vi "Choreo_DifferentialSample_Interpolate.vi"(9 "TimeStamp":dbl, 10 "endValueSample":T1={"timestamp"=-999.0, "x"=0.0, "y"=0.0, "heading"=0.0, "velocityL"=0.0, "velocityR"=0.0, "angularVelocity"=0.0, "accelL"=0.0, "accelR"=0.0, "accelAngular"=0.0, "forceL"=0.0, "forceR"=0.0}, 11 "ChoreoDifferentialSample":T1={"timestamp"=-999.0, "x"=0.0, "y"=0.0, "heading"=0.0, "velocityL"=0.0, "velocityR"=0.0, "angularVelocity"=0.0, "accelL"=0.0, "accelR"=0.0, "accelAngular"=0.0, "forceL"=0.0, "forceR"=0.0}) -> (3 "InterpolatedSample":T1={"timestamp"=-999.0, "x"=0.0, "y"=0.0, "heading"=0.0, "velocityL"=0.0, "velocityR"=0.0, "angularVelocity"=0.0, "accelL"=0.0, "accelR"=0.0, "accelAngular"=0.0, "forceL"=0.0, "forceR"=0.0})   [LabVIEW 2019, in "ChoreoLib.lvlib"]
doc: "Interpolate between two Differential Trajectory Samples.\n\nInputs:\n -- ChoreoDifferentialSample - cluster - Differential sample.\n -- endChoreoDifferentialSample - cluster - The end Differential sample\n -- TimeStamp - double - desired time stamp\n\nOutputs:\n -- InterpolatedSample - cluster - Interpolated Differential sample."
uses:
  ChoreoLib.lvlib
  TypeDef/ChoreoDifferentialSample.ctl
  <vilib>/Rock Robotics/WPI/ThirdParty/JAS_Junk/TrajLib/MathUtil_Clamp.vi
  Choreo_DifferentialSample_IntegrateFunction.vi
  <vilib>/Rock Robotics/WPI/ThirdParty/JAS_Junk/TrajLib/Trajectory_Library.lvlib
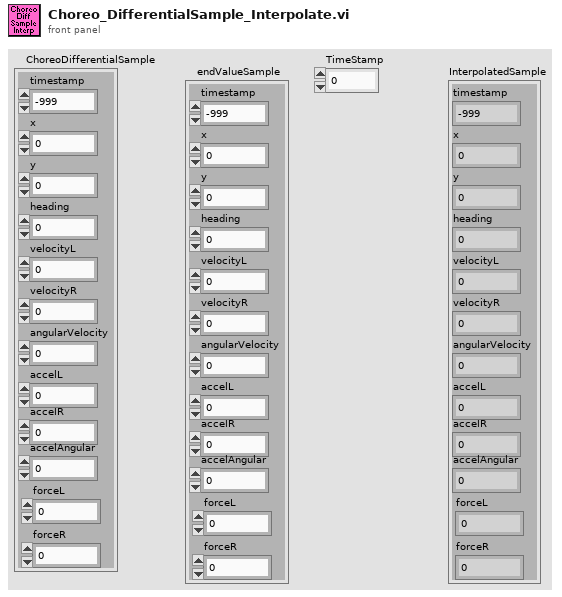
[diagram p1: front panel]
types:
  T1 = typedef "ChoreoLib.lvlib/ChoreoDifferentialSample.ctl" = cluster{"timestamp":dbl, "x":dbl, "y":dbl, "heading":dbl, "velocityL":dbl, "velocityR":dbl, "angularVelocity":dbl, "accelL":dbl, "accelR":dbl, "accelAngular":dbl, "forceL":dbl, "forceR":dbl}
  T2 = typedef "NI_Matrix.lvlib/RealMatrix.ctl" = dbl[][]
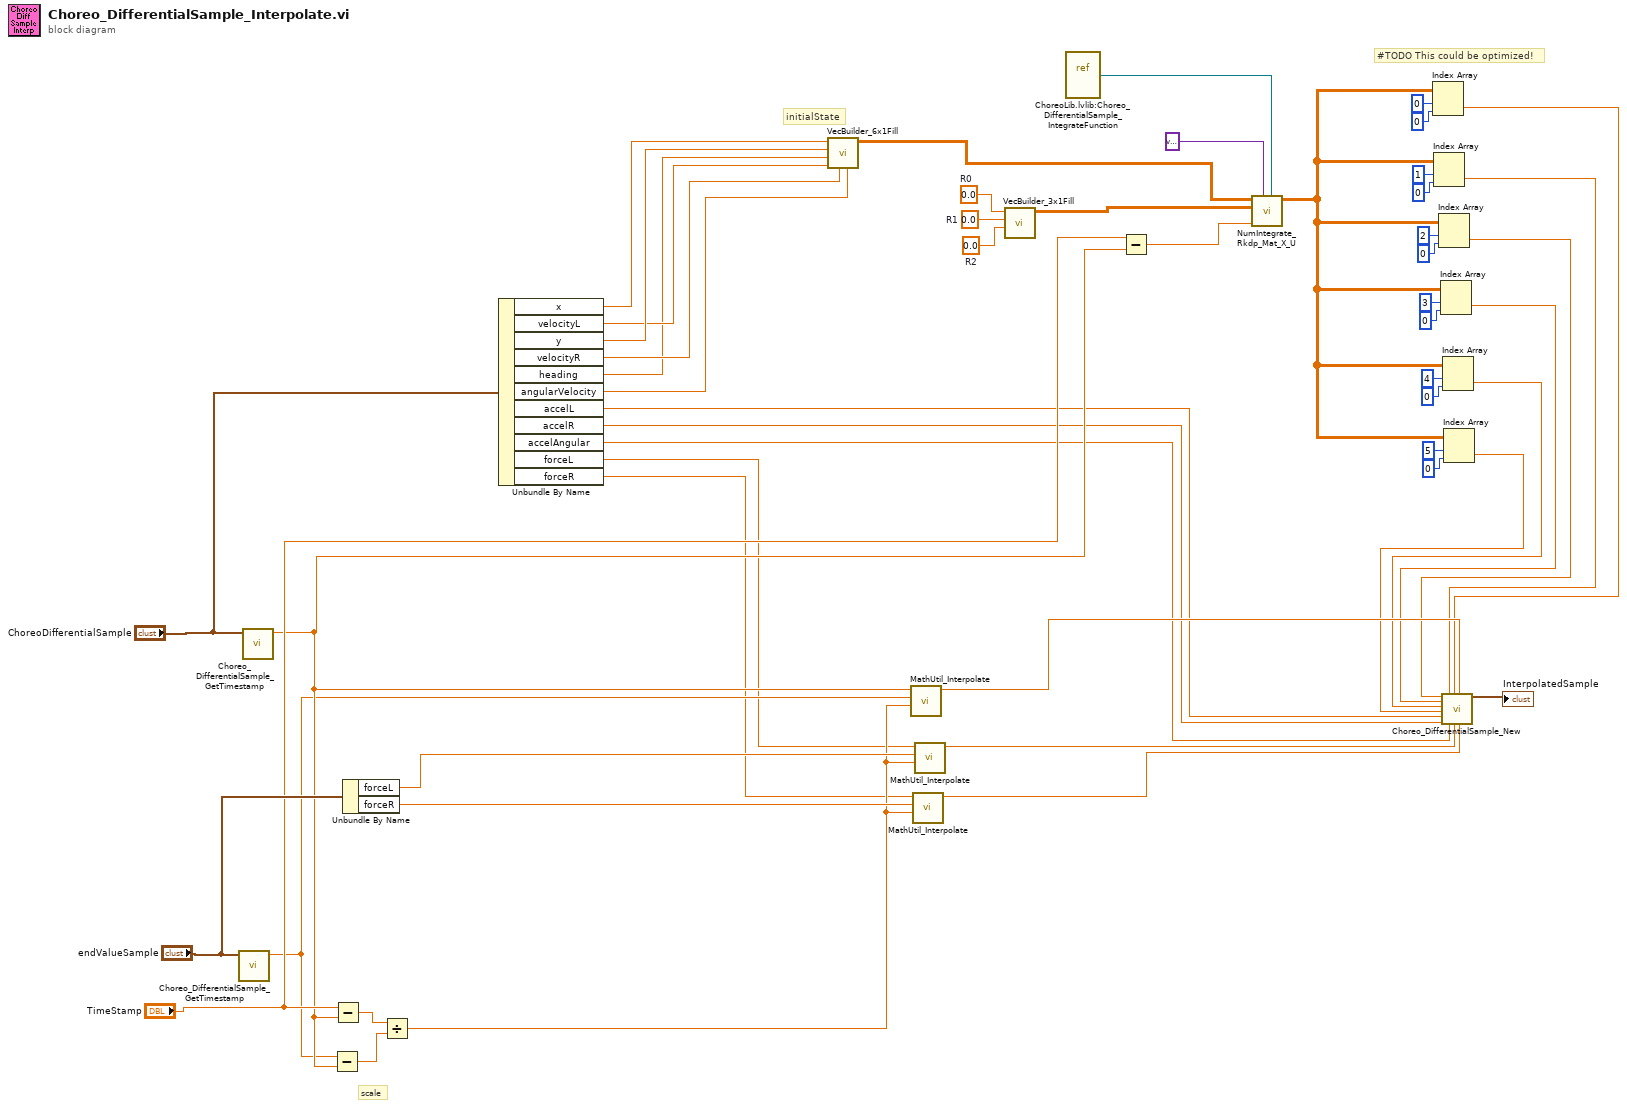
[diagram p0: block diagram]
diagram:
  w35 = 0.0  # R2
  w34 = 0.0  # R1
  w33 = 0.0  # R0
  # "#TODO This could be optimized!"
  # "initialState"
  # "scale"
  n1 = call "Choreo_DifferentialSample_GetTimestamp.vi"("ChoreoDifferentialSample"="endValueSample") -> ("Timestamp"=w28:dbl)  [unwired: 10 in]
  n2 = call "Choreo_DifferentialSample_GetTimestamp.vi"("ChoreoDifferentialSample"="ChoreoDifferentialSample") -> ("Timestamp"=w29:dbl)  [unwired: 10 in]
  n3 = Subtract(x=w28, y=w29) -> (x-y=w51:dbl)
  n4 = Subtract(x="TimeStamp", y=w29) -> (x-y=w52:dbl)
  n5 = Unbundle By Name("endValueSample") -> ("forceL"=w47:dbl, "forceR"=w44:dbl)
  n6 = Divide(x=w52, y=w51) -> (x/y=w27:dbl)
  n7 = Unbundle By Name("ChoreoDifferentialSample") -> ("x"=w43:dbl, "velocityL"=w41:dbl, "y"=w42:dbl, "velocityR"=w40:dbl, "heading"=w6:dbl, "angularVelocity"=w39:dbl, "accelL"=w3:dbl, "accelR"=w2:dbl, "accelAngular"=w1:dbl, "forceL"=w5:dbl, "forceR"=w4:dbl)
  n8 = call <vilib>:"VecBuilder_6x1Fill.vi"("R5"=w39, "R4"=w40, "R3"=w41, "R2"=w6, "R1"=w42, "R0"=w43) -> ("output matrix"=w36:T2)  [unwired: 5 in]
  n9 = call <vilib>:"MathUtil_Interpolate.vi"("T"=w27, "EndValue"=w28, "StartValue"=w29) -> ("InterpolatedValue"=w26:dbl)  [unwired: 8 in]
  n10 = call <vilib>:"MathUtil_Interpolate.vi"("T"=w27, "EndValue"=w44, "StartValue"=w4) -> ("InterpolatedValue"=w46:dbl)  [unwired: 8 in]
  n11 = call <vilib>:"MathUtil_Interpolate.vi"("T"=w27, "EndValue"=w47, "StartValue"=w5) -> ("InterpolatedValue"=w45:dbl)  [unwired: 8 in]
  n12 = call <vilib>:"VecBuilder_3x1Fill.vi"("R2"=w35, "R1"=w34, "R0"=w33) -> ("output matrix"=w32:T2)  [unwired: 8 in]
  n13 = vi-ref "ChoreoLib.lvlib:Choreo_DifferentialSample_IntegrateFunction.vi"() -> (w38:refnum<vi>)
  n14 = Subtract(x="TimeStamp", y=w29) -> (x-y=w30:dbl)
  n15 = call <vilib>:"NumIntegrate_Rkdp_Mat_X_U.vi"("Func_X_U_Extra"=w38, "PassedData"=variant, "dT_Seconds"=w30, "U"=w32, "X"=w36) -> ("Return X"=w11:T2)  [unwired: 4 in, 2 out]
  n16 = Index Array(array=w11, index (row)=0, index (col)=0) -> (element=w13:dbl)
  n17 = Index Array(array=w11, index (row)=1, index (col)=0) -> (element=w12:dbl)
  n18 = Index Array(array=w11, index (row)=2, index (col)=0) -> (element=w10:dbl)
  n19 = Index Array(array=w11, index (row)=3, index (col)=0) -> (element=w9:dbl)
  n20 = Index Array(array=w11, index (row)=4, index (col)=0) -> (element=w8:dbl)
  n21 = Index Array(array=w11, index (row)=5, index (col)=0) -> (element=w7:dbl)
  n22 = call "Choreo_DifferentialSample_New.vi"("heading"=w10, "velocityL"=w9, "velocityR"=w8, "angularVelocity"=w7, "accelL"=w3, "accelR"=w2, "y"=w12, "accelAngular"=w1, "x"=w13, "forceL"=w45, "timestamp"=w26, "forceR"=w46) -> ("ChoreoDifferentialSample"=→"InterpolatedSample":T1)  [unwired: 7 in]
